vi "TAT_Varient Creater.vi"(8 "error in (no error)":errorcluster) -> (0 "error out":errorcluster)   [LabVIEW 2017]
uses:
  <vilib>/Utility/config.llb/NI_LVConfig.lvlib
panel:
  in  "TEST STEPS":T1 {"CHANNEL 3"."Output USB Port Vtg Tolerance" format="%#_g  V"; "CHANNEL 3"."Output Port Vtg" format="%#_g  V"; "CHANNEL 3"."Current" format="%#_g mA"; "CHANNEL 3"."Current Tolerance" format="%#_g mA"; "CHANNEL 3"."Input Vtg Tolerance" format="%#_g  V"; "CHANNEL 3"."Input Vtg" format="%#_g  V"; "CHANNEL 2"."Output USB Port Vtg Tolerance" format="%#_g  V"; "CHANNEL 2"."Output Port Vtg" format="%#_g  V"; "CHANNEL 2"."Current" format="%#_g mA"; "CHANNEL 2"."Current Tolerance" format="%#_g mA"; "CHANNEL 2"."Input Vtg Tolerance" format="%#_g  V"; "CHANNEL 2"."Input Vtg" format="%#_g  V"; "CHANNEL 1"."Output USB Port Vtg Tolerance" format="%#_g  V"; "CHANNEL 1"."Output Port Vtg" format="%#_g  V"; "CHANNEL 1"."Current" format="%#_g mA"; "CHANNEL 1"."Current Tolerance" format="%#_g mA"; "CHANNEL 1"."Input Vtg Tolerance" format="%#_g  V"; "CHANNEL 1"."Input Vtg" format="%#_g  V"}
  in  "Cancle 2":bool
  in  "Delete Button":bool
  in  "Cancle":bool
  in  "Save Button":bool
  in  "HOME":bool
  in  "MODEL NAME":string(combo)
  # "RECIPE CREATOR"
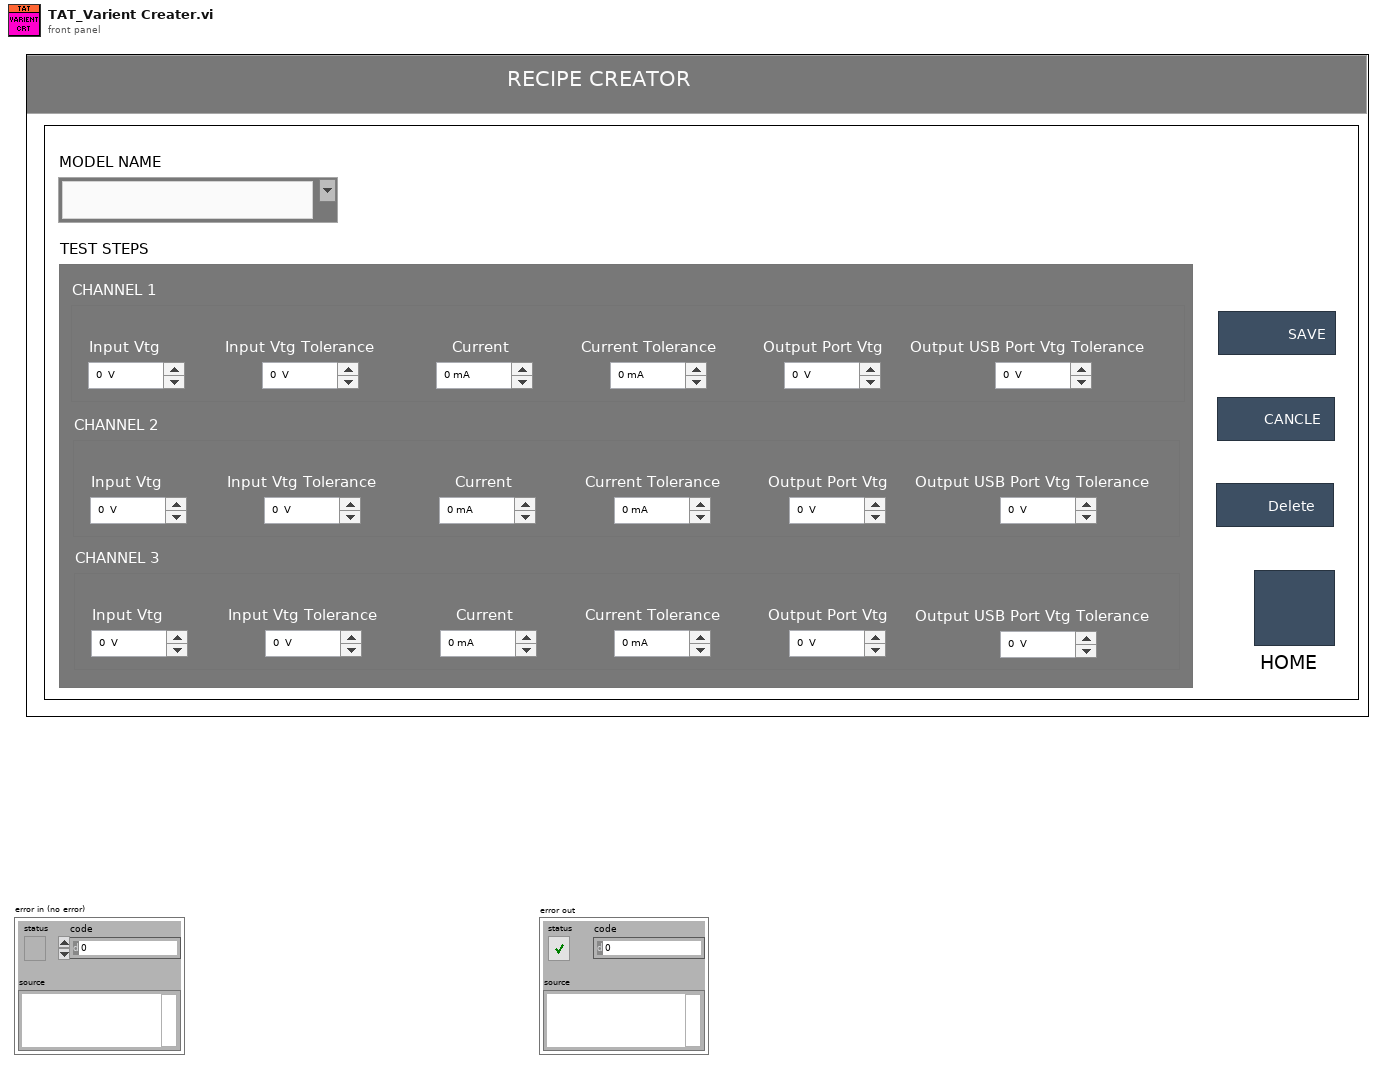
[diagram p1: front panel]
types:
  T1 = cluster{"CHANNEL 1":cluster{"Input Vtg":dbl, "Input Vtg Tolerance":dbl, "Current Tolerance":dbl, "Current":dbl, "Output Port Vtg":dbl, "Output USB Port Vtg Tolerance":dbl}, "CHANNEL 2":cluster{"Input Vtg":dbl, "Input Vtg Tolerance":dbl, "Current Tolerance":dbl, "Current":dbl, "Output Port Vtg":dbl, "Output USB Port Vtg Tolerance":dbl}, "CHANNEL 3":cluster{"Input Vtg":dbl, "Input Vtg Tolerance":dbl, "Current Tolerance":dbl, "Current":dbl, "Output Port Vtg":dbl, "Output USB Port Vtg Tolerance":dbl}}
  T2 = cluster{"CHANNEL 1":cluster{"Input Vtg":dbl, "Input Vtg Tolerance":dbl, "Current Tolerance":dbl, "Current":dbl, "Output Port Vtg":dbl, "Output USB Port \nVtg Tolerance":dbl}, "CHANNEL 2":cluster{"Input Vtg":dbl, "Input Vtg Tolerance":dbl, "Current Tolerance":dbl, "Current":dbl, "Output Port Vtg":dbl, "Output USB Port \nVtg Tolerance":dbl}, "CHANNEL 3":cluster{"Input Vtg":dbl, "Input Vtg Tolerance":dbl, "Current Tolerance":dbl, "Current":dbl, "Output Port Vtg":dbl, "Output USB Port \nVtg Tolerance":dbl}}
  T3 = enum32{"invalid app kind", "Development System", "Run Time System", "Student Edition", "Embedded LabVIEW", "Evaluation", "Custom"}
  T4 = typedef "NI_LVConfig.lvlib/Config Data RefNum.ctl" = refnum<k1>
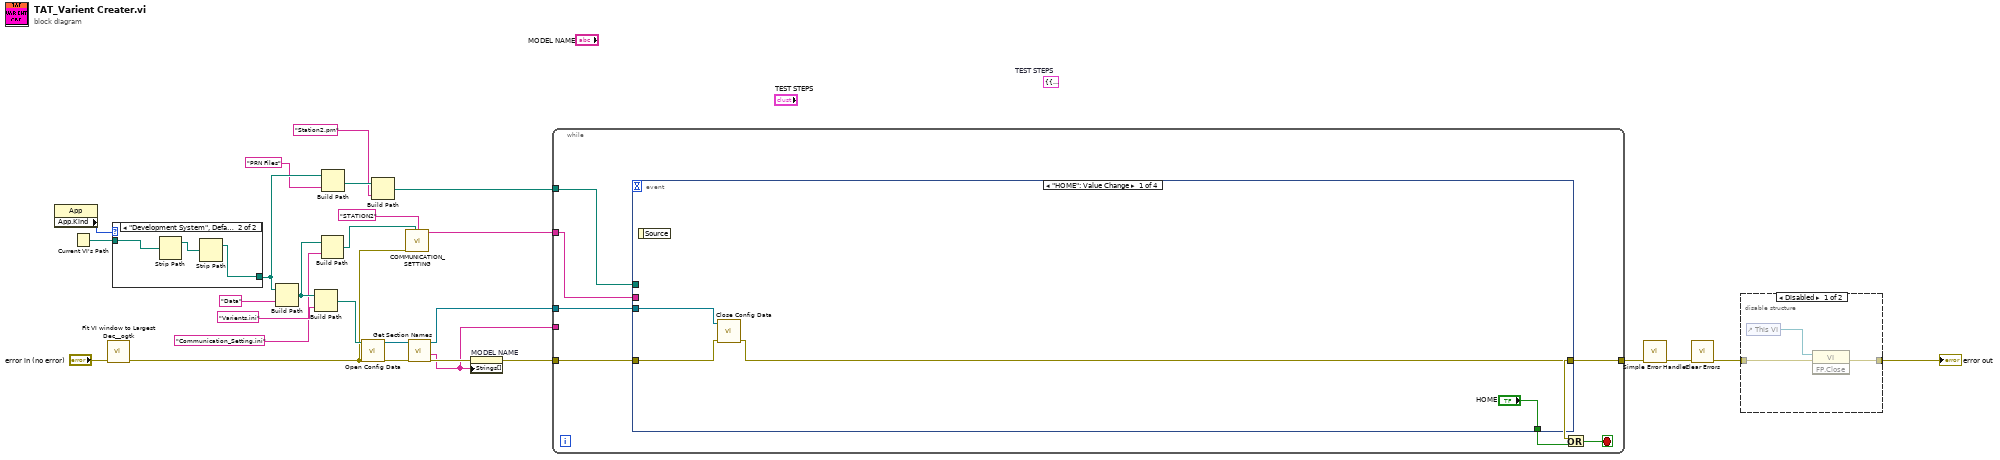
[diagram p0: block diagram]
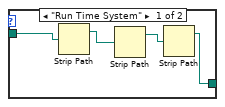
[diagram p3: hidden frame]
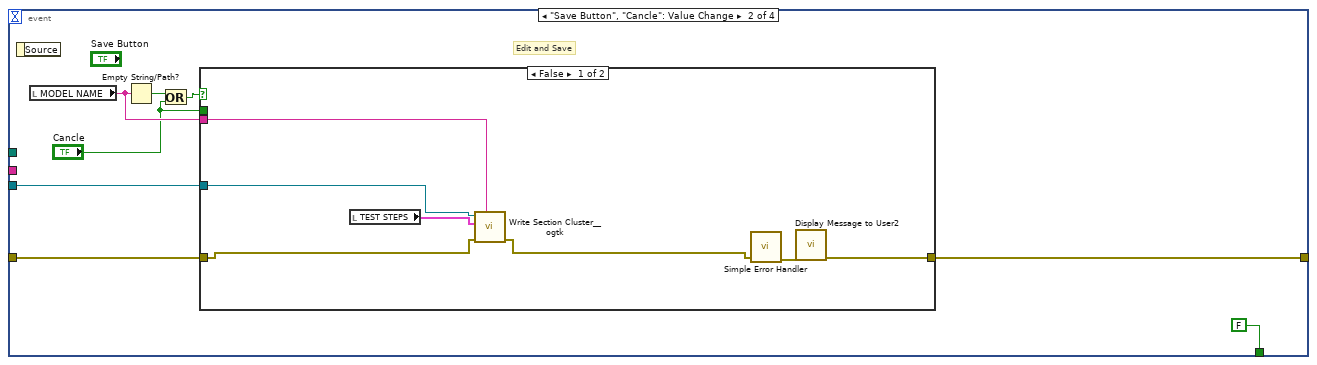
[diagram p4: hidden frame]
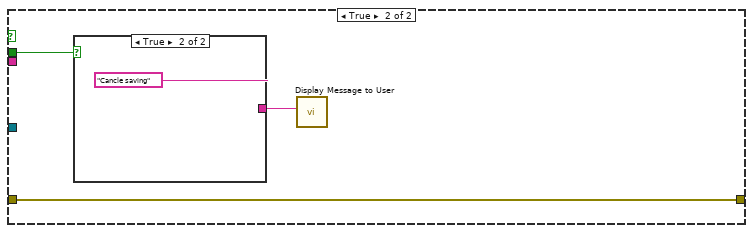
[diagram p5: hidden frame]
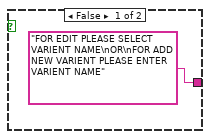
[diagram p6: hidden frame]
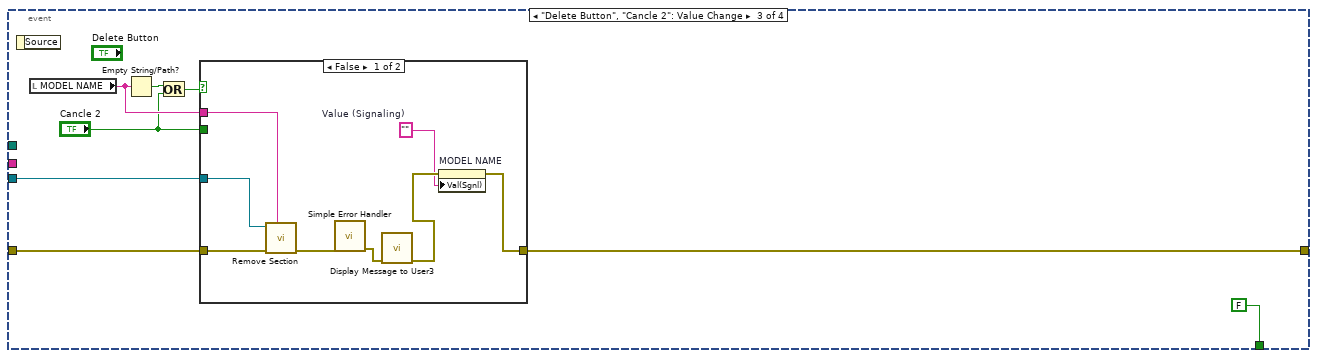
[diagram p7: hidden frame]
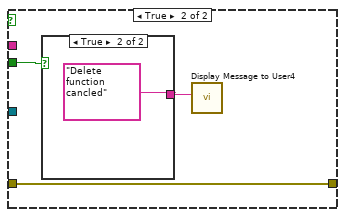
[diagram p8: hidden frame]
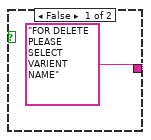
[diagram p9: hidden frame]
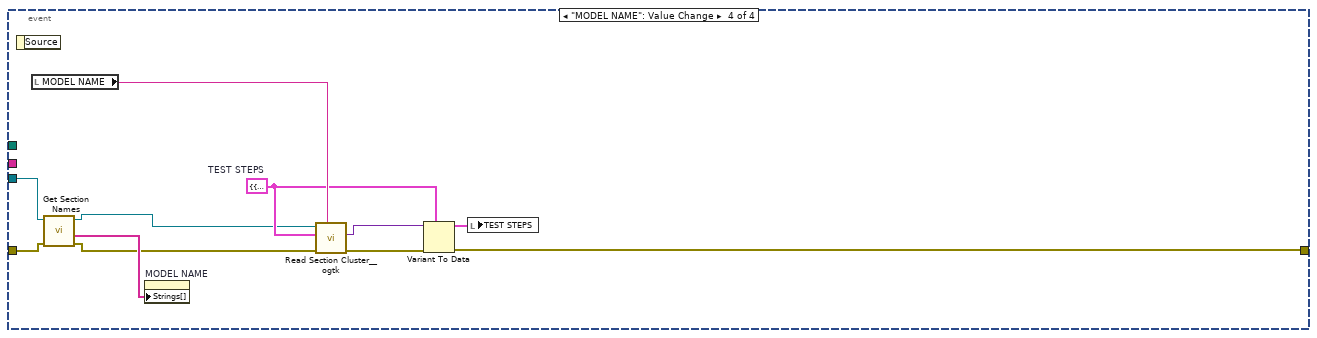
[diagram p10: hidden frame]
diagram:
  (unwired) T2 {"CHANNEL 1"={"Input Vtg"=0.0, "Input Vtg Tolerance"=0.0, "Current Tolerance"=-1.0, "Current"=-1.0, "Output Port Vtg"=-1.0, "Output USB Port \nVtg Tolerance"=-1.0}, "CHANNEL 2"={"Input Vtg"=0.0, "Input Vtg Tolerance"=0.0, "Current Tolerance"=-1.0, "Current"=-1.0, "Output Port Vtg"=-1.0, "Output USB Port \nVtg Tolerance"=-1.0}, "CHANNEL 3"={"Input Vtg"=0.0, "Input Vtg Tolerance"=0.0, "Current Tolerance"=-1.0, "Current"=-1.0, "Output Port Vtg"=-1.0, "Output USB Port \nVtg Tolerance"=-1.0}}  # TEST STEPS
  n1 = property class="App"() -> ("App.Kind"=w22:T3)  [unwired: 2 in, 2 out]
  n2 = Current VI's Path() -> (path=w23:path)
  n3 = call <userlib>:"Fit VI window to Largest Dec__ogtk.vi"("error in (no error)"="error in (no error)") -> ("error out"=w11:errorcluster)  [unwired: 5 in, 1 out]
  n4 = case shown="\"Development System\", Default" w22 {
    tunnel: w23 -> [w29 w33]
    tunnel: [w28 w32] -> w5
    frame "Run Time System" {
      n5 = Strip Path(path=w29) -> (stripped path=w31:path)  [unwired: 1 out]
      n6 = Strip Path(path=w31) -> (stripped path=w30:path)  [unwired: 1 out]
      n7 = Strip Path(path=w30) -> (stripped path=w28:path)  [unwired: 1 out]
    }
    frame "Development System", Default {
      n8 = Strip Path(path=w33) -> (stripped path=w34:path)  [unwired: 1 out]
      n9 = Strip Path(path=w34) -> (stripped path=w32:path)  [unwired: 1 out]
    }
  }
  n10 = Build Path(base path=w5, name or relative path="Data") -> (appended path=w10:path)
  n11 = Build Path(base path=w10, name or relative path="Varients.ini") -> (appended path=w21:path)
  n12 = Build Path(base path=w10, name or relative path="Communication_Setting.ini") -> (appended path=w7:path)
  n13 = Build Path(base path=w5, name or relative path="PRN Files") -> (appended path=w3:path)
  n14 = call <vilib>:"Open Config Data.vi"("error in (no error)"=w11, "configuration file path"=w21) -> ("error out"=w17:errorcluster, "refnum"=w18:T4)  [unwired: 7 in, 1 out]
  n15 = Build Path(base path=w3, name or relative path="Station2.prn") -> (appended path=w1:path)
  n16 = call "COMMUNICATION_SETTING.vi"("communication path"=w7, "error in"=w11, "STATION"="STATION2") -> ("PRINT_COM"=w6:string)  [unwired: 6 in, 2 out]
  n17 = call <vilib>:"Get Section Names.vi"("error in (no error)"=w17, "refnum"=w18) -> ("error out"=w16:errorcluster, "section names"=w13:string[], "refnum out"=w15:T4)  [unwired: 7 in]
  n18 = property on="MODEL NAME" class="CmbBox"(error in=w16, "Strings[]"=w13) -> (error out=w14:errorcluster)  [unwired: 1 in, 1 out]
  n19 = while {
    tunnel: w14 -> [w40]
    tunnel: [w38] -> w24
    tunnel: w15 -> [w37]
    tunnel: w13 -> [_]
    tunnel: w6 -> [w36]
    tunnel: w1 -> [w35]
    stop <- w39 stop-if-true
    n20 = event shown="[0] \"HOME\": Value Change" {
      selector: _ -> [_ _ _ _]
      dyn-events: _ -> [_ _ _ _]
      timeout: _ -> [_ _ _ _]
      tunnel: ["HOME" FALSE ("stop") FALSE ("stop") _] -> w41
      tunnel: w40 -> [w44 w51 w71 w88]
      tunnel: [w43 w46 w66 w92] -> w38
      tunnel: w37 -> [w42 w52 w72 w90]
      tunnel: w36 -> [_ _ _ _]
      tunnel: w35 -> [_ _ _ _]
      event "HOME": Value Change {
        n21 = event-data() -> ()  [unwired: 1 in, 1 out]
        n22 = call <vilib>:"Close Config Data.vi"("error in (no error)"=w44, "refnum"=w42) -> ("error out"=w43:errorcluster)  [unwired: 8 in, 1 out]
      }
      event "Save Button", "Cancle": Value Change {
        # "Edit and Save"
        n23 = event-data() -> ()  [unwired: 1 in, 1 out]
        n24 = local read "MODEL NAME"() -> (w50:string)
        n25 = Empty String/Path?(string/path=w50) -> (empty?=w49:bool)
        n26 = Or(x=w49, y="Cancle") -> (x .or. y?=w48:bool)
        n27 = case shown="False" w48 {
          tunnel: w51 -> [w56 w63]
          tunnel: [w54 w63] -> w46
          tunnel: w52 -> [w57 _]
          tunnel: w50 -> [w59 _]
          tunnel: "Cancle" -> [_ w61]
          frame False {
            n28 = local read "TEST STEPS"() -> (w58:T1)
            n29 = call <userlib>:"Write Section Cluster__ogtk.vi"("section (optional)"=w59, "error in (no error)"=w56, "Section Formatted Cluster"=w58, "refnum"=w57) -> ("error out"=w55:errorcluster)  [unwired: 6 in, 1 out]
            n30 = call <vilib>:"Simple Error Handler.vi"("error in (no error)"=w55) -> ("error out"=w60:errorcluster)  [unwired: 4 in, 4 out]
            n31 = call "Display Message to User2"("error in (no error)"=w60) -> ("error out"=w54:errorcluster)  [unwired: 9 in, 1 out]
          }
          frame True {
            n32 = case shown="True" w61 {
              tunnel: ["FOR EDIT PLEASE SELECT VARIENT NAME\nOR\nFOR ADD NEW VARIENT PLEASE ENTER VARIENT NAME" "Cancle saving"] -> w62
              frame False {
              }
              frame True {
              }
            }
            n33 = call "Display Message to User"("Message"=w62) -> ()  [unwired: 9 in, 2 out]
          }
        }
      }
      event "Delete Button", "Cancle 2": Value Change {
        n34 = event-data() -> ()  [unwired: 1 in, 1 out]
        n35 = local read "MODEL NAME"() -> (w70:string)
        n36 = Empty String/Path?(string/path=w70) -> (empty?=w69:bool)
        n37 = Or(x=w69, y="Cancle 2") -> (x .or. y?=w68:bool)
        n38 = case shown="False" w68 {
          tunnel: w71 -> [w78 w84]
          tunnel: [w76 w84] -> w66
          tunnel: w72 -> [w79 _]
          tunnel: w70 -> [w80 _]
          tunnel: "Cancle 2" -> [_ w83]
          frame False {
            w74 = ""  # Value (Signaling)
            n39 = call <vilib>:"Remove Section.vi"("section"=w80, "error in (no error)"=w78, "refnum"=w79) -> ("error out"=w77:errorcluster)  [unwired: 6 in, 2 out]
            n40 = call <vilib>:"Simple Error Handler.vi"("error in (no error)"=w77) -> ("error out"=w81:errorcluster)  [unwired: 4 in, 4 out]
            n41 = call "Display Message to User3"("error in (no error)"=w81) -> ("error out"=w75:errorcluster)  [unwired: 9 in, 1 out]
            n42 = property on="MODEL NAME" class="CmbBox"(error in=w75, "Val(Sgnl)"=w74) -> (error out=w76:errorcluster)  [unwired: 1 in, 1 out]
          }
          frame True {
            n43 = case shown="True" w83 {
              tunnel: ["FOR DELETE PLEASE SELECT VARIENT NAME" "Delete function cancled"] -> w82
              frame False {
              }
              frame True {
              }
            }
            n44 = call "Display Message to User4"("Message"=w82) -> ()  [unwired: 9 in, 2 out]
          }
        }
      }
      event "MODEL NAME": Value Change {
        w96 = T2 {"CHANNEL 1"={"Input Vtg"=0.0, "Input Vtg Tolerance"=0.0, "Current Tolerance"=-1.0, "Current"=-1.0, "Output Port Vtg"=-1.0, "Output USB Port \nVtg Tolerance"=-1.0}, "CHANNEL 2"={"Input Vtg"=0.0, "Input Vtg Tolerance"=0.0, "Current Tolerance"=-1.0, "Current"=-1.0, "Output Port Vtg"=-1.0, "Output USB Port \nVtg Tolerance"=-1.0}, "CHANNEL 3"={"Input Vtg"=0.0, "Input Vtg Tolerance"=0.0, "Current Tolerance"=-1.0, "Current"=-1.0, "Output Port Vtg"=-1.0, "Output USB Port \nVtg Tolerance"=-1.0}}  # TEST STEPS
        n45 = event-data() -> ()  [unwired: 1 in, 1 out]
        n46 = local read "MODEL NAME"() -> (w97:string)
        n47 = call <vilib>:"Get Section Names.vi"("error in (no error)"=w88, "refnum"=w90) -> ("error out"=w87:errorcluster, "section names"=w91:string[], "refnum out"=w89:T4)  [unwired: 7 in]
        n48 = property on="MODEL NAME" class="CmbBox"("Strings[]"=w91) -> ()  [unwired: 2 in, 2 out]
        n49 = call <userlib>:"Read Section Cluster__ogtk.vi"("section (optional)"=w97, "error in (no error)"=w87, "Section Formatted Cluster Type"=w96, "refnum"=w89) -> ("error out"=w93:errorcluster, "Section Formatted Cluster"=w95:variant)  [unwired: 3 in, 3 out]
        n50 = Variant To Data(error in=w93, type=w96, Variant=w95) -> (data=w94:T2, error out=w92:errorcluster)
        n51 = local write "TEST STEPS"(w94) -> ()
      }
    }
    n52 = Or(x=w38, y=w41) -> (x .or. y?=w39:bool)
  }
  n53 = call <vilib>:"Simple Error Handler.vi"("error in (no error)"=w24) -> ("error out"=w27:errorcluster)  [unwired: 4 in, 4 out]
  n54 = call <vilib>:"Clear Errors.vi"("error in (no error)"=w27) -> ("error out"=w26:errorcluster)  [unwired: 5 in, 1 out]
  n55 = disable-structure shown="Disabled" {
    disable-tunnel: w26 -> [w100 w101]
    disable-tunnel: [w99 w101] -> w25
    frame Disabled {
      n56 = control-ref of="This VI"() -> (w98:refnum<vi>)
      n57 = invoke class="VI" method="FP.Close"(reference=w98, error in=w100) -> (error out=w99:errorcluster)  [unwired: 1 in, 2 out]
    }
    frame Enabled {
    }
  }
  "error out" <- w25
